vi "Test ISA010_module API.vi"() -> ()   [LabVIEW 2017]
doc: "ISA010_module API Tester."
uses:
  ISA010_module.lvlib
panel:
  in  "cofig json":string="{\"MQTT\":\"{\\\"client\\\":\\\"ISAMQTTDriver1\\\",\\\"broker\\\":{\\\"address\\\":\\\"192.168.20.249\\\",\\\"port\\\":1883,\\\"connTimeout\\\":5000,\\\"writeTimeout\\\":5000,\\\"readTimeout\\\":5000,\\\"subTimeout\\\":5000},\\\"connFlags\\\":{\\\"reserved\\\":false,\\\"clean session\\\":true,\\\"will flag\\\":false,\\\"willQOS\\\":\\\"\\\",\\\"will retain\\\":false,\\\"password\\\":false,\\\"user name\\\":false},\\\"User Info\\\":{\\\"User Name\\\":\\\"\\\",\\\"Password\\\":\\\"\\\"}}\",\"MOXA\":\"{\\\"Plugin\\\":\\\"MOXAIP\\\",\\\"IP\\\":\\\"192.168.20.118\\\",\\\"Port\\\":4001}\"}"
  in  "config":bool
  in  "KAAWAR_go":bool
  in  "KASAWAR":bool
  in  "dkgGo":bool
  in  "DKG":bool
  in  "serviceMode":bool
  in  "pwmval":u8
  in  "pwm":bool
  in  "state":bool
  in  "Run as Singleton?":bool
  in  "Show Block Diagram":bool
  in  "Refresh Modules":bool
  out "Active Modules":string[](array[string])
  in  "Stop Module":bool
  in  "Select Module":i32(ring)=-1 caption="Select Module\nTo send Request to" items=["All"=-1]
  in  "Run New Module":bool
  in  "Hide Module Panel":bool
  in  "Show Module Panel":bool
  out "Status":string
  # "This VI tests the API for the Module."
  # "{\"MQTT\":\"{\\\"Broker\\\":{\\\"IP\\\":\\\"192.168.20.249\\\",\\\"port\\\":1883,\\\"connTimeout\\\":3000,\\\"writeTimeout\\\":3000,\\\"readTimeout\\\":3000,\\\"subTimeout\\\":3000},\\\"Connect Flags\\\":{\\\"reserved\\\":false,\\\"clean session\\\":false,\\\"will flag\\\":true,\\\"willQOS\\\":\\\"At least once\\\",\\\"will retain\\\":true,\\\"password\\\":false,\\\"user name\\\":false},\\\"Keep Alive\\\":5000,\\\"Client Info\\\":{\\\"ClientId\\\":\\\"ISADriver101047\\\",\\\"Will Topic\\\":\\\"ISA010/Online\\\",\\\"Will Message\\\":\\\"flase\\\",\\\"User Name\\\":\\\"\\\",\\\"Password\\\":\\\"\\\"}}\",\"MOXA\":\"{\\n  \\\"Plugin\\\":\\\"MOXAIP\\\",\\n  \\\"IP\\\":\\\"192.168.20.118\\\",\\n  \\\"Port\\\":4001\\n}\"}"
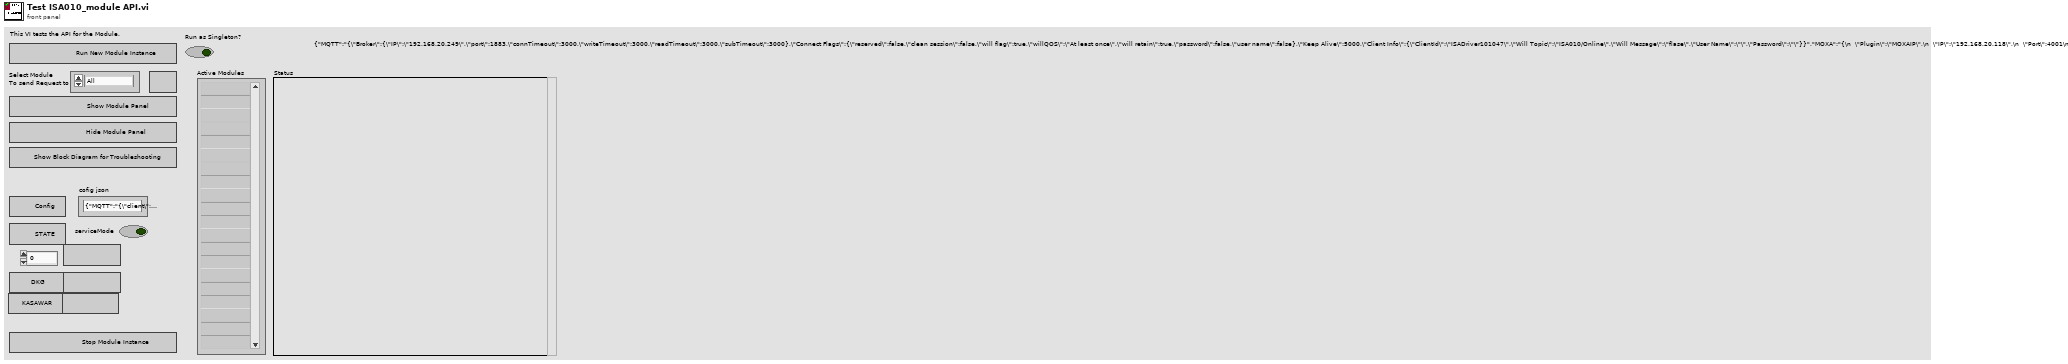
[diagram p1: front panel]
types:
  T1 = typedef "ISA010_module.lvlib/Broadcast Events--cluster.ctl" = cluster{"Module Did Init":refnum<user-event>, "Status Updated":refnum<user-event>, "Error Reported":refnum<user-event>, "Module Did Stop":refnum<user-event>, "Update Module Execution Status":refnum<user-event>, "ISA010State":refnum<user-event>}
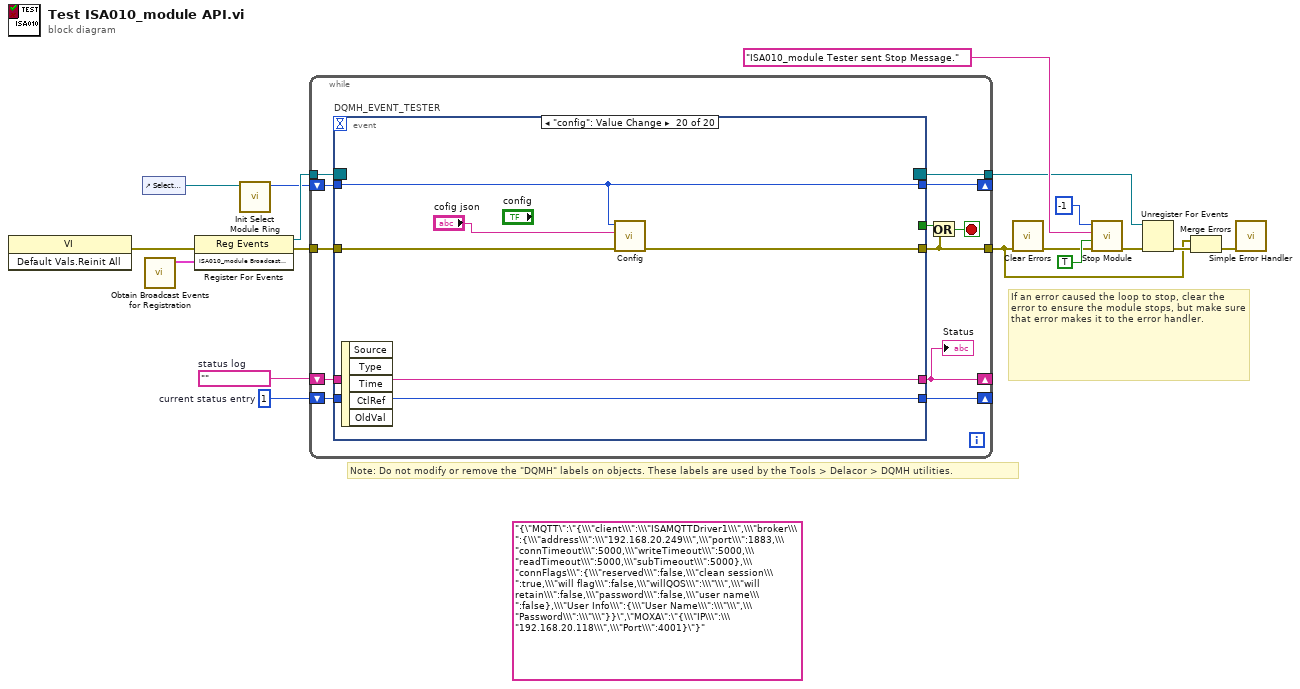
[diagram p0: block diagram]
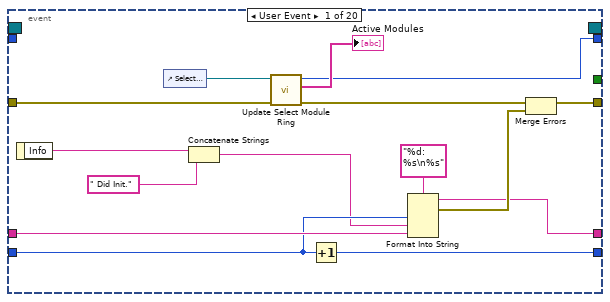
[diagram p2: hidden frame]
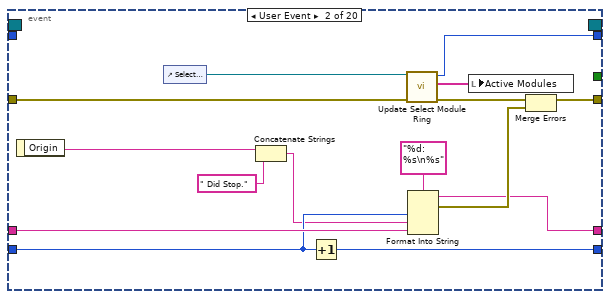
[diagram p3: hidden frame]
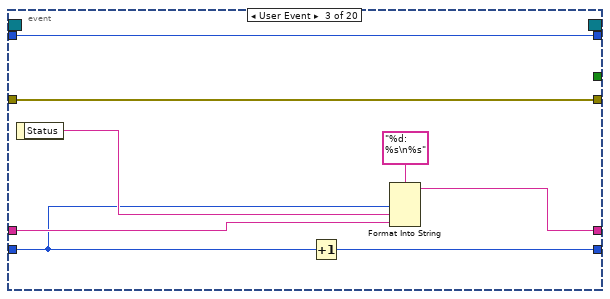
[diagram p4: hidden frame]
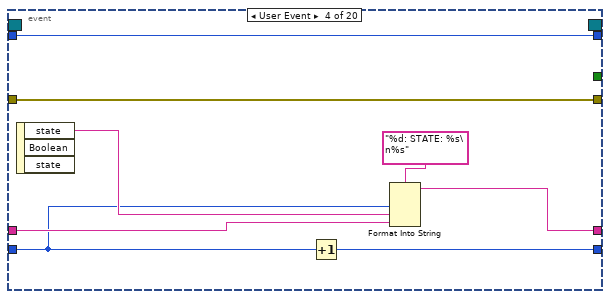
[diagram p5: hidden frame]
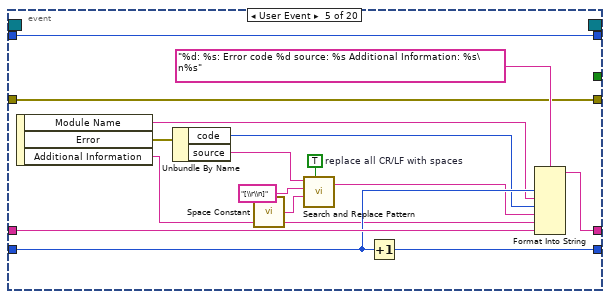
[diagram p6: hidden frame]
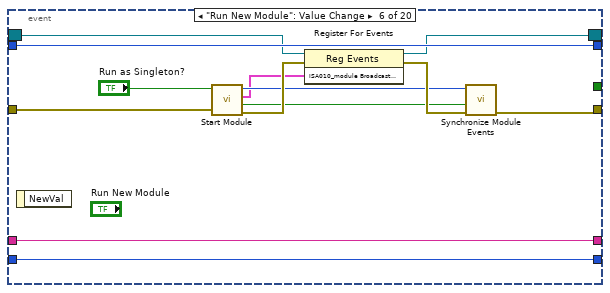
[diagram p7: hidden frame]
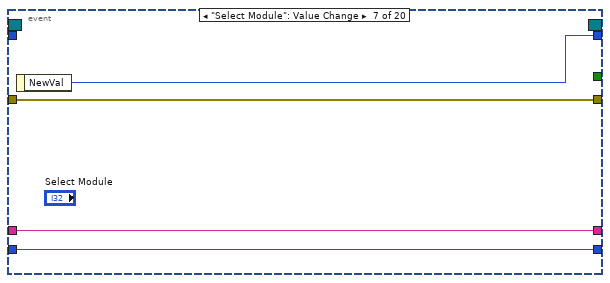
[diagram p8: hidden frame]
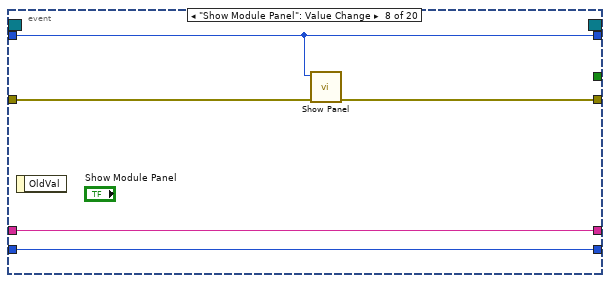
[diagram p9: hidden frame]
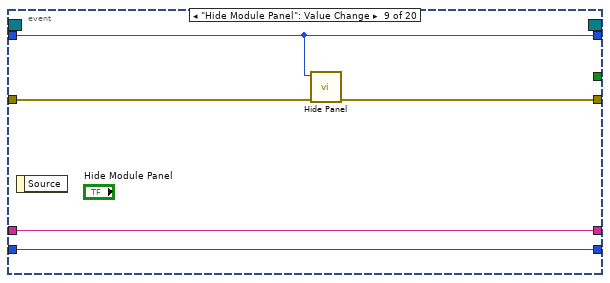
[diagram p10: hidden frame]
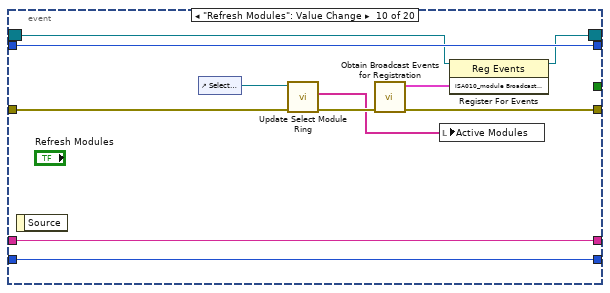
[diagram p11: hidden frame]
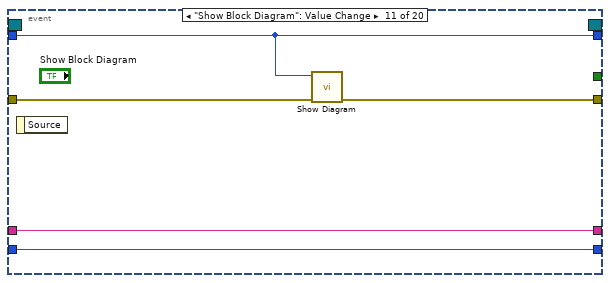
[diagram p12: hidden frame]
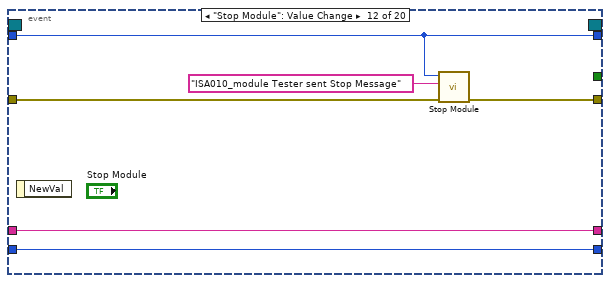
[diagram p13: hidden frame]
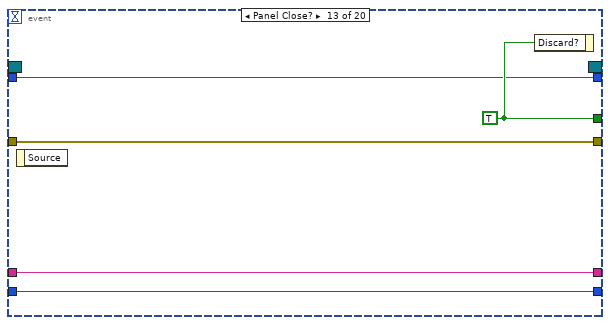
[diagram p14: hidden frame]
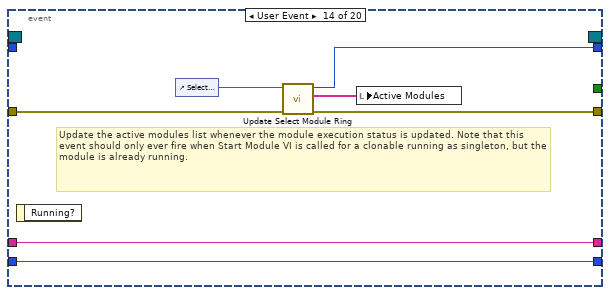
[diagram p15: hidden frame]
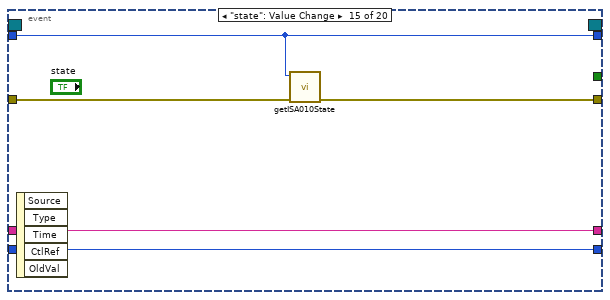
[diagram p16: hidden frame]
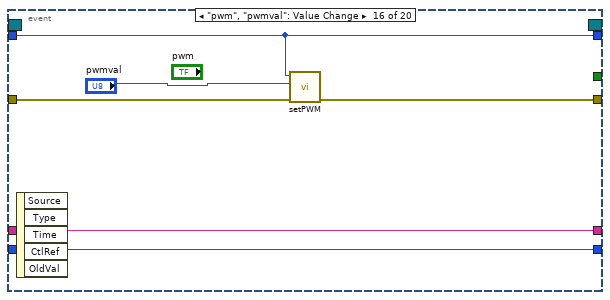
[diagram p17: hidden frame]
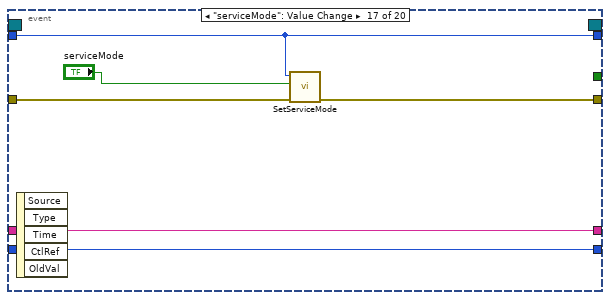
[diagram p18: hidden frame]
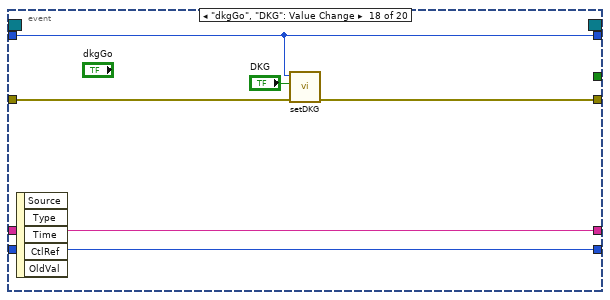
[diagram p19: hidden frame]
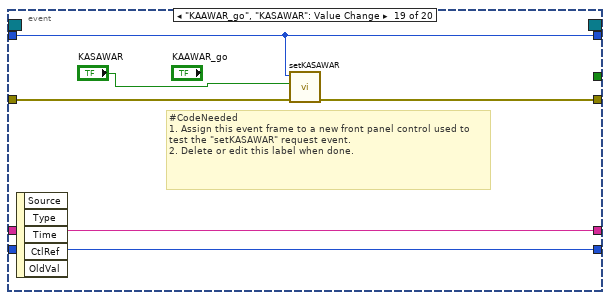
[diagram p20: hidden frame]
diagram:
  (unwired) "{\"MQTT\":\"{\\\"client\\\":\\\"ISAMQTTDriver1\\\",\\\"broker\\\":{\\\"address\\\":\\\"192.168.20.249\\\",\\\"port\\\":1883,\\\"connTimeout\\\":5000,\\\"writeTimeout\\\":5000,\\\"readTimeout\\\":5000,\\\"subTimeout\\\":5000},\\\"connFlags\\\":{\\\"reserved\\\":false,\\\"clean session\\\":true,\\\"will flag\\\":false,\\\"willQOS\\\":\\\"\\\",\\\"will retain\\\":false,\\\"password\\\":false,\\\"user name\\\":false},\\\"User Info\\\":{\\\"User Name\\\":\\\"\\\",\\\"Password\\\":\\\"\\\"}}\",\"MOXA\":\"{\\\"IP\\\":\\\"192.168.20.118\\\",\\\"Port\\\":4001}\"}"
  w13 = 1  # current status entry
  w14 = ""  # status log
  # "If an error caused the loop to stop, clear the error to ensure the module stops, but make sure that error makes it to the error handler."
  # "Note: Do not modify or remove the \"DQMH\" labels on objects. These labels are used by the Tools > Delacor > DQMH utilities."
  n1 = invoke class="VI" method="Default Vals.Reinit All"() -> (error out=w6:errorcluster)  [unwired: 3 in, 2 out]
  n2 = control-ref of="Select Module"() -> (w11:refnum<vi>)
  n3 = call "Obtain Broadcast Events for Registration.vi"() -> ("ISA010_module Broadcast Events"=w10:T1)  [unwired: 10 in, 1 out]
  n4 = register-events(error in=w6, w10) -> (reference out=w17:refnum<event-registration>, error out=w9:errorcluster)  [unwired: 1 in]
  n5 = call "Init Select Module Ring.vi"("Select Module Ring Ref"=w11) -> ("Value for All Modules"=w12:i32)  [unwired: 8 in, 2 out]
  n6 = while {
    tunnel: w17 -> [w29]
    tunnel: [w18] -> w1
    tunnel: w9 -> [w27]
    shift-right: [w23] -> _
    shift-left: w14 -> [w25]
    shift-right: [w24] -> _
    shift-left: w13 -> [w26]
    shift-right: [w20] -> _
    shift-left: w12 -> [w21]
    tunnel: [w19] -> w5
    stop <- w22 stop-if-true
    n7 = event "DQMH_EVENT_TESTER" shown="[19] \"config\": Value Change" {
      selector: w29 -> [_ _ _ _ _ w98 _ _ _ w124 _ _ _ _ _ _ _ _ _ _]
      dyn-events: [_ _ _ _ _ w97 _ _ _ w123 _ _ _ _ _ _ _ _ _ _] -> w19
      timeout: _ -> [_ _ _ _ _ _ _ _ _ _ _ _ _ _ _ _ _ _ _ _]
      tunnel: [_ _ _ _ _ _ _ _ _ _ _ _ w145 _ _ _ _ _ _ _] -> w28
      tunnel: [w33 w51 w67 w75 w81 w96 w108 w112 w117 w120 w131 w136 w144 w148 w154 w160 w166 w172 w178 w184] -> w18
      tunnel: w27 -> [w35 w53 w67 w75 w81 w99 w108 w113 w118 w125 w134 w137 w144 w149 w157 w163 w169 w175 w181 w187]
      tunnel: w26 -> [w41 w56 w60 w68 w87 w101 w106 w110 w115 w128 w132 w139 w142 w151 w155 w161 w167 w173 w179 w185]
      tunnel: w25 -> [w42 w57 w63 w71 w89 w102 w107 w111 w116 w129 w133 w140 w143 w152 w156 w162 w168 w174 w180 w186]
      tunnel: [w39 w54 w64 w72 w84 w102 w107 w111 w116 w129 w133 w140 w143 w152 w156 w162 w168 w174 w180 w186] -> w23
      tunnel: [w40 w55 w66 w74 w90 w101 w106 w110 w115 w128 w132 w139 w142 w151 w155 w161 w167 w173 w179 w185] -> w24
      tunnel: w21 -> [_ _ w61 w69 w91 w100 _ w109 w114 w127 w130 w138 w141 _ w153 w158 w164 w170 w177 w182]
      tunnel: [w30 w48 w61 w69 w91 w100 w105 w109 w114 w127 w130 w138 w141 w147 w153 w158 w164 w170 w177 w182] -> w20
      event User Event {
        n8 = event-data() -> ("Info"=w38:string)  [unwired: 1 in]
        n9 = control-ref of="Select Module"() -> (w32:refnum<vi>)
        n10 = Concatenate Strings(w38, " Did Init.") -> (w37:string)
        n11 = call "Update Select Module Ring.vi"("error in (no error)"=w35, "Select Module Ring Ref"=w32) -> ("error out"=w34:errorcluster, "Active Modules (Array)"=→"Active Modules":string[], "New Module Ring Value"=w30:i32)  [unwired: 7 in]
        n12 = Increment(x=w41) -> (x+1=w40:i32)
        n13 = Format Into String(format string="%d: %s\n%s", w41, w37, w42) -> (resulting string=w39:string, error out=w44:errorcluster)  [unwired: 2 in]
        n14 = Merge Errors(w34, w44) -> (w33:errorcluster)
      }
      event User Event {
        n15 = event-data() -> ("Origin"=w46:string)  [unwired: 1 in]
        n16 = control-ref of="Select Module"() -> (w50:refnum<vi>)
        n17 = Concatenate Strings(w46, " Did Stop.") -> (w45:string)
        n18 = Increment(x=w56) -> (x+1=w55:i32)
        n19 = call "Update Select Module Ring.vi"("error in (no error)"=w53, "Select Module Ring Ref"=w50) -> ("error out"=w52:errorcluster, "Active Modules (Array)"=w49:string[], "New Module Ring Value"=w48:i32)  [unwired: 7 in]
        n20 = Format Into String(format string="%d: %s\n%s", w56, w45, w57) -> (resulting string=w54:string, error out=w59:errorcluster)  [unwired: 2 in]
        n21 = local write "Active Modules"(w49) -> ()
        n22 = Merge Errors(w52, w59) -> (w51:errorcluster)
      }
      event User Event {
        n23 = event-data() -> ("Status"=w62:string)  [unwired: 1 in]
        n24 = Increment(x=w60) -> (x+1=w66:i32)
        n25 = Format Into String(format string="%d: %s\n%s", w60, w62, w63) -> (resulting string=w64:string)  [unwired: 2 in, 1 out]
      }
      event User Event {
        n26 = event-data() -> ("state"=w70:string)  [unwired: 1 in, 2 out]
        n27 = Increment(x=w68) -> (x+1=w74:i32)
        n28 = Format Into String(format string="%d: STATE: %s\n%s", w68, w70, w71) -> (resulting string=w72:string)  [unwired: 2 in, 1 out]
      }
      event User Event {
        w85 = TRUE  # replace all CR/LF with spaces
        n29 = event-data() -> ("Module Name"=w79:string, "Error"=w78:errorcluster, "Additional Information"=w76:string)  [unwired: 1 in]
        n30 = Unbundle By Name(w78) -> ("code"=w80:i32, "source"=w82:string)
        n31 = call <vilib>:"Space Constant.vi"() -> ("String"=w86:string)
        n32 = call <vilib>:"Search and Replace Pattern.vi"("string"=w82, "regular expression (\"\")"="[\\r\\n]" ("regular expression (\"\")"), "replace string (\"\")"=w86, "replace all? (F)"=w85) -> ("result string"=w83:string)  [unwired: 1 in, 1 out]
        n33 = Increment(x=w87) -> (x+1=w90:i32)
        n34 = Format Into String(format string="%d: %s: Error code %d source: %s Additional Information: %s\n%s", w87, w79, w80, w83, w76, w89) -> (resulting string=w84:string)  [unwired: 2 in, 1 out]
      }
      event "Run New Module": Value Change {
        n35 = event-data() -> ()  [unwired: 1 in, 1 out]
        n36 = call "Start Module.vi"("error in (no error)"=w99, "Run as Singleton? (F)"="Run as Singleton?") -> ("error out"=w103:errorcluster, "Wait for Event Sync?"=w94:bool, "ISA010_module Broadcast Events"=w93:T1, "Module ID"=w95:i32)  [unwired: 6 in]
        n37 = register-events(reference=w98, error in=w103, w93) -> (reference out=w97:refnum<event-registration>, error out=w104:errorcluster)
        n38 = call "Synchronize Module Events.vi"("error in (no error)"=w104, "Wait for Event Sync?"=w94, "Module ID"=w95) -> ("error out"=w96:errorcluster)  [unwired: 7 in, 1 out]
      }
      event "Select Module": Value Change {
        n39 = event-data() -> ("NewVal"=w105:i32)  [unwired: 1 in]
      }
      event "Show Module Panel": Value Change {
        n40 = event-data() -> ()  [unwired: 1 in, 1 out]
        n41 = call "Show Panel.vi"("error in (no error)"=w113, "Module ID"=w109) -> ("error out"=w112:errorcluster)  [unwired: 9 in]
      }
      event "Hide Module Panel": Value Change {
        n42 = event-data() -> ()  [unwired: 1 in, 1 out]
        n43 = call "Hide Panel.vi"("error in (no error)"=w118, "Module ID"=w114) -> ("error out"=w117:errorcluster)  [unwired: 9 in]
      }
      event "Refresh Modules": Value Change {
        n44 = event-data() -> ()  [unwired: 1 in, 1 out]
        n45 = control-ref of="Select Module"() -> (w126:refnum<vi>)
        n46 = call "Update Select Module Ring.vi"("error in (no error)"=w125, "Select Module Ring Ref"=w126) -> ("error out"=w121:errorcluster, "Active Modules (Array)"=w119:string[])  [unwired: 7 in, 1 out]
        n47 = call "Obtain Broadcast Events for Registration.vi"("error in (no error)"=w121) -> ("error out"=w120:errorcluster, "ISA010_module Broadcast Events"=w122:T1)  [unwired: 9 in]
        n48 = local write "Active Modules"(w119) -> ()
        n49 = register-events(reference=w124, w122) -> (reference out=w123:refnum<event-registration>)  [unwired: 1 in, 1 out]
      }
      event "Show Block Diagram": Value Change {
        n50 = event-data() -> ()  [unwired: 1 in, 1 out]
        n51 = call "Show Diagram.vi"("error in (no error)"=w134, "Module ID"=w130) -> ("error out"=w131:errorcluster)  [unwired: 9 in]
      }
      event "Stop Module": Value Change {
        n52 = event-data() -> ()  [unwired: 1 in, 1 out]
        n53 = call "Stop Module.vi"("error in (no error)"=w137, "Origin"="ISA010_module Tester sent Stop Message", "Module ID"=w138) -> ("error out"=w136:errorcluster)  [unwired: 8 in]
      }
      event Panel Close? {
        w145 = TRUE ("Discard?")
        n54 = event-data() -> ()  [unwired: 1 in, 1 out]
        n55 = event-data("Discard?"=w145) -> ()  [unwired: 1 in, 1 out]
      }
      event User Event {
        # "Update the active modules list whenever the module execution status is updated. Note that this event should only ever fire when Start Module VI is called for a clonable running as singleton, but the module is already running."
        n56 = event-data() -> ()  [unwired: 1 in, 1 out]
        n57 = control-ref of="Select Module"() -> (w150:refnum<vi>)
        n58 = call "Update Select Module Ring.vi"("error in (no error)"=w149, "Select Module Ring Ref"=w150) -> ("error out"=w148:errorcluster, "Active Modules (Array)"=w146:string[], "New Module Ring Value"=w147:i32)  [unwired: 7 in]
        n59 = local write "Active Modules"(w146) -> ()
      }
      event "state": Value Change {
        n60 = event-data() -> ()  [unwired: 1 in, 5 out]
        n61 = call "getISA010State.vi"("error in (no error)"=w157, "Module ID"=w153) -> ("error out"=w154:errorcluster)  [unwired: 9 in]
      }
      event "pwm", "pwmval": Value Change {
        n62 = event-data() -> ()  [unwired: 1 in, 5 out]
        n63 = call "setPWM.vi"("error in (no error)"=w163, "PWM"="pwmval", "Module ID"=w158) -> ("error out"=w160:errorcluster)  [unwired: 8 in]
      }
      event "serviceMode": Value Change {
        n64 = event-data() -> ()  [unwired: 1 in, 5 out]
        n65 = call "SetServiceMode.vi"("error in (no error)"=w169, "SET"="serviceMode", "Module ID"=w164) -> ("error out"=w166:errorcluster)  [unwired: 8 in]
      }
      event "dkgGo", "DKG": Value Change {
        n66 = event-data() -> ()  [unwired: 1 in, 5 out]
        n67 = call "setDKG.vi"("error in (no error)"=w175, "DKG"="DKG", "Module ID"=w170) -> ("error out"=w172:errorcluster)  [unwired: 8 in]
      }
      event "KAAWAR_go", "KASAWAR": Value Change {
        # "#CodeNeeded\n1. Assign this event frame to a new front panel control used to test the \"setKASAWAR\" request event.\n2. Delete or edit this label when done."
        n68 = event-data() -> ()  [unwired: 1 in, 5 out]
        n69 = call "setKASAWAR.vi"("error in (no error)"=w181, "KASAWAR"="KASAWAR", "Module ID"=w177) -> ("error out"=w178:errorcluster)  [unwired: 8 in]
      }
      event "config": Value Change {
        n70 = event-data() -> ()  [unwired: 1 in, 5 out]
        n71 = call "Config.vi"("error in (no error)"=w187, "ConfigJson"="cofig json", "Module ID"=w182) -> ("error out"=w184:errorcluster)  [unwired: 8 in]
      }
    }
    "Status" <- w23
    n72 = Or(x=w28, y=w18) -> (x .or. y?=w22:bool)
  }
  n73 = call <vilib>:"Clear Errors.vi"("error in (no error)"=w1) -> ("error out"=w3:errorcluster)  [unwired: 5 in, 1 out]
  n74 = call "Stop Module.vi"("error in (no error)"=w3, "Wait for Module to stop? (F)"=TRUE ("Wait for Module to stop?"), "Origin"="ISA010_module Tester sent Stop Message.", "Module ID"=-1 ("Stop all")) -> ("error out"=w15:errorcluster)  [unwired: 7 in]
  n75 = Unregister For Events(event registration refnum=w5, error in=w15) -> (error out=w16:errorcluster)
  n76 = Merge Errors(w1, w16) -> (w2:errorcluster)
  n77 = call <vilib>:"Simple Error Handler.vi"("error in (no error)"=w2) -> ()  [unwired: 4 in, 5 out]
